vi "Calibration Models Comparison.vi"() -> ()   [LabVIEW 2014]
doc: "This example compares measurement accuracies obtained using different types of calibration models. Several calibration templates have been learned offline using the Calibration Training interface.\n\nFor each of the calibration models, the example locates the part in the image and measures its height along 50 search lines. The process is repeated for 25 different locations in the image using the same part. The example computes the average and standard deviation of the measurement set and plots the measurement distribution in a histogram."
uses:
  <vilib>/Utility/miscctls.llb/LVRowAndColumnUnsignedTypeDef.ctl
  <vilib>/Analysis/NI_AALBase.lvlib
  <vilib>/vision/NI_Vision_Development_Module.lvlib
panel:
  in  "Tab Control":enum32{"Part Image", "Calibration Grid Image"}(tab)
  out "Test Image":T1(plugin-control)
  out "Calibration Grid":T1(plugin-control)
  in  "Stop Button":bool
  out "Measurement Distribution Graph":T2(graph)
  in  "Results":i32(listbox)
  # "Overview: Compares accuracy and speed of the different spatial calibration methods.\nRequirements: NI Vision Development Module\nInstructions: Run the VI."
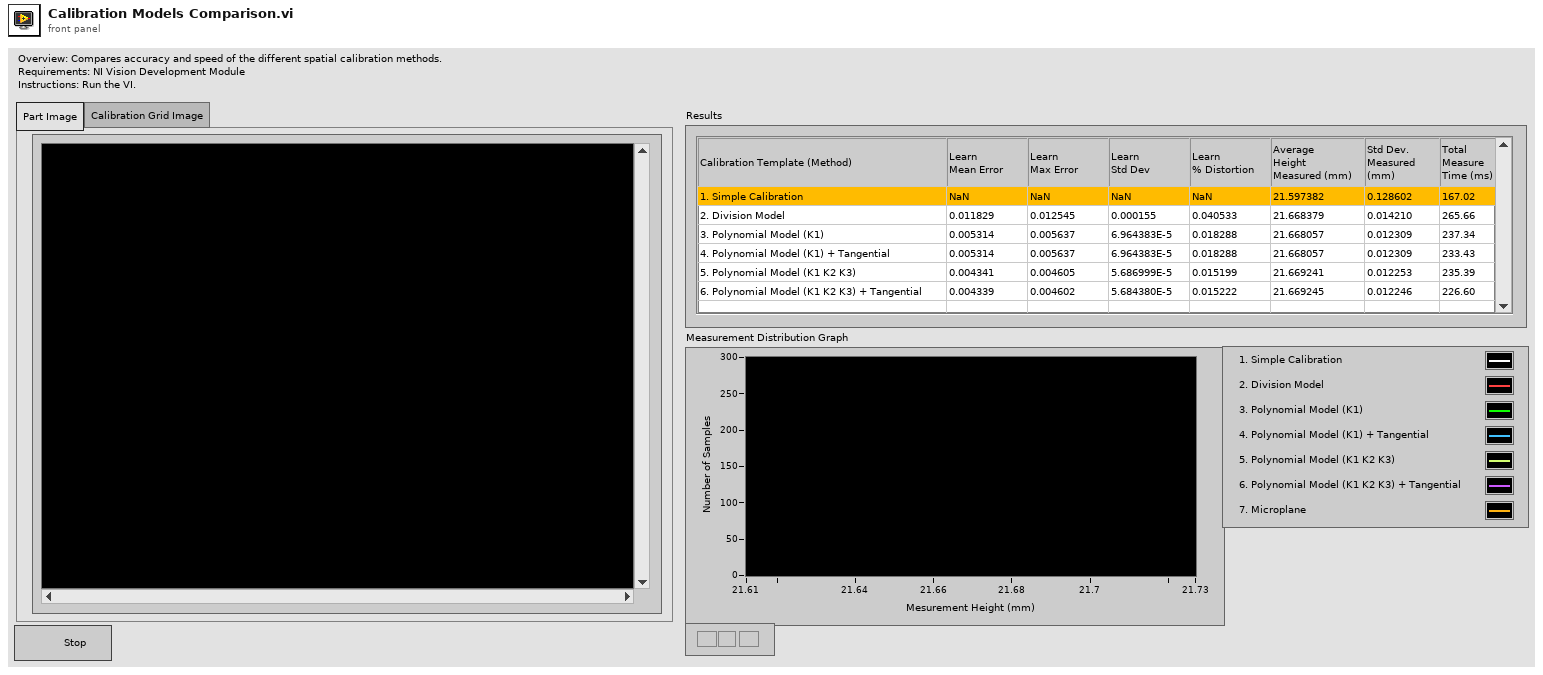
[diagram p1: front panel]
types:
  T1 = typedef "IMAQ Image.ctl" = refnum<image>
  T2 = cluster{"X Values":dbl[], "Histogram: h(x)":i32[]}[]
  T3 = typedef "LVRowAndColumnUnsignedTypeDef.ctl" = cluster{"Row":u32, "Column":u32}
  T4 = typedef "Correction Learn Setup.ctl" = cluster{"Method":u32, "Distortion":T5, "Corrected Image Scaling":u32, "Corrected Image Learn ROI":u32, "Learn Correction Table?":bool}
  T5 = typedef "Distortion Model Types.ctl" = i32
  T6 = typedef "Error Statistics.ctl" = cluster{"Mean Error":dbl, "Maximum Error":dbl, "Standard Deviation":dbl, "% Distortion":dbl}
  T7 = cluster{"X Values":dbl[], "Histogram: h(x)":i32[]}
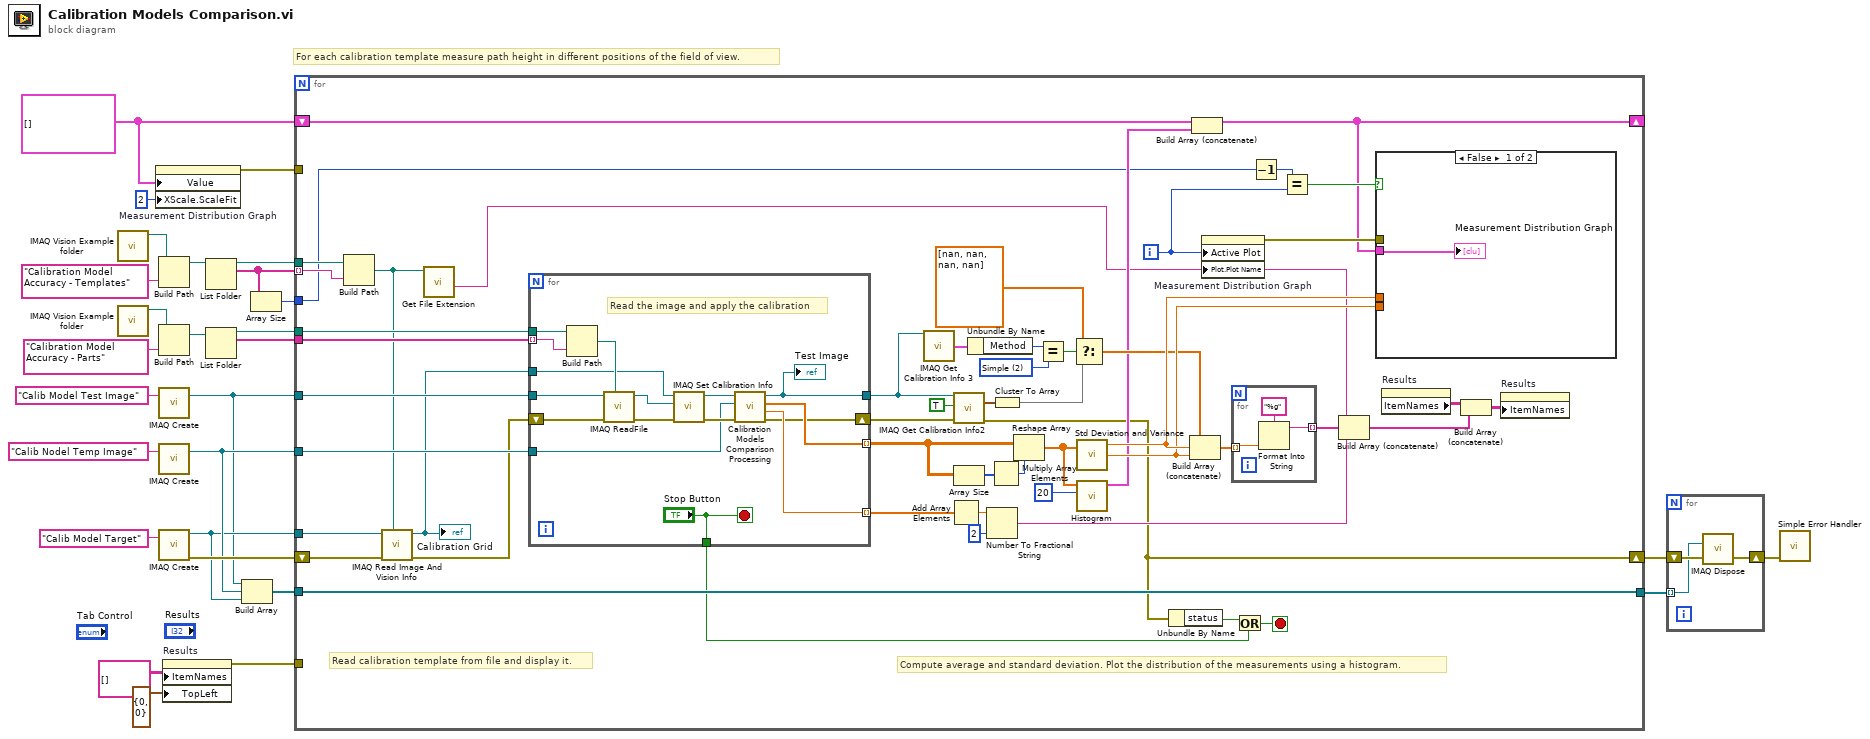
[diagram p0: block diagram]
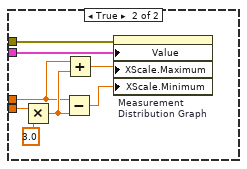
[diagram p2: hidden frame]
diagram:
  w17 = T2 [] ("Measurement Distribution")
  # "For each calibration template measure path height in different positions of the field of view."
  n1 = call "IMAQ Vision Example folder.vi"() -> ("Example Image Path"=w14:path)  [unwired: 11 in]
  n2 = call "IMAQ Vision Example folder.vi"() -> ("Example Image Path"=w12:path)  [unwired: 11 in]
  n3 = property on="Measurement Distribution Graph" class="XYGraph (strict)"("Value"=w17, "XScale.ScaleFit"=u8 2 ("X Scale.Scale Fit")) -> (error out=w16:errorcluster)  [unwired: 2 in, 1 out]
  n4 = Build Path(base path=w14, name or relative path="Calibration Model Accuracy - Templates") -> (appended path=w13:path)
  n5 = Build Path(base path=w12, name or relative path="Calibration Model Accuracy - Parts") -> (appended path=w11:path)
  n6 = call "IMAQ Create"("Image Name"="Calib Model Test Image") -> ("New Image"=w6:T1)  [unwired: 3 in, 2 out]
  n7 = call "IMAQ Create"("Image Name"="Calib Nodel Temp Image") -> ("New Image"=w9:T1)  [unwired: 3 in, 2 out]
  n8 = call "IMAQ Create"("Image Name"="Calib Model Target") -> ("New Image"=w8:T1, "error out"=w23:errorcluster)  [unwired: 3 in, 1 out]
  n9 = property on="Results" class="MCListbox (strict)"("ItemNames"=string[][] [] ("Item Names"), "TopLeft"=T3 {"Row"=0, "Column"=0} ("Top Left Visible Cell")) -> (error out=w20:errorcluster)  [unwired: 2 in, 1 out]
  n10 = List Folder(path=w13) -> (path out=w22:path, filenames=w2:string[])  [unwired: 1 in, 4 out]
  n11 = List Folder(path=w11) -> (path out=w27:path, filenames=w26:string[])  [unwired: 1 in, 4 out]
  n12 = Build Array(w6, w9, w8) -> (w7:T1[])
  n13 = Array Size(array=w2) -> (size(s)=w1:i32)
  n14 = for {
    tunnel: w27 -> [w77]
    tunnel: w26 -> [w76]
    tunnel: w6 -> [w75]
    tunnel: w9 -> [w74]
    tunnel: w8 -> [w80]
    tunnel: w22 -> [w78]
    tunnel: w2 -> [w72] mode=indexing
    tunnel: w20 -> [_]
    shift-right: [w50] -> _
    shift-left: w17 -> [w70]
    tunnel: w16 -> [_]
    shift-right: [w35] -> w5
    shift-left: w23 -> [w79]
    tunnel: w7 -> [w47]
    tunnel: [w47] -> w4
    tunnel: w1 -> [w36]
    i -> [w71]
    stop <- w33 stop-if-true
    w42 = u32 2 items=["Perspective", "Microplane", "Simple", "Corrected", "None"] ("Method")
    # "Compute average and standard deviation. Plot the distribution of the measurements using a histogram."
    # "Read calibration template from file and display it."
    n15 = Build Path(base path=w78, name or relative path=w72) -> (appended path=w31:path)
    n16 = call "IMAQ Read Image And Vision Info"("File Path"=w31, "error in (no error)"=w79, "Image"=w80) -> ("error out"=w73:errorcluster, "Image Out"=w48:T1)  [unwired: 1 in, 6 out]
    "Calibration Grid" <- w48
    n17 = call <vilib>:"Get File Extension.vi"("file"=w31) -> ("filename without extension"=w30:string)  [unwired: 7 in, 3 out]
    n18 = for {
      tunnel: w77 -> [w108]
      tunnel: w76 -> [w107] mode=indexing
      tunnel: w75 -> [w106]
      tunnel: w74 -> [w93]
      tunnel: [w104] -> w46 mode=indexing
      tunnel: w48 -> [w97]
      tunnel: ["Stop Button"] -> w32
      tunnel: [w103] -> w68 mode=indexing
      shift-right: [w94] -> w49
      shift-left: w73 -> [w100]
      tunnel: [w95] -> w45
      stop <- "Stop Button" stop-if-true
      # "Read the image and apply the calibration"
      n19 = Build Path(base path=w108, name or relative path=w107) -> (appended path=w105:path)
      n20 = call "IMAQ ReadFile"("File Path"=w105, "error in (no error)"=w100, "Image"=w106) -> ("error out"=w99:errorcluster, "Image Out"=w101:T1)  [unwired: 2 in, 5 out]
      n21 = call "IMAQ Set Calibration Info"("error in (no error)"=w99, "Image Dst"=w101, "Image Src"=w97) -> ("error out"=w98:errorcluster, "Calibrated Image"=w96:T1)  [unwired: 1 in, 6 out]
      n22 = call "Calibration Models Comparison Processing.vi"("error in (no error)"=w98, "Temp Image"=w93, "Test Image"=w96) -> ("error out"=w94:errorcluster, "Elapsed Time (ms)"=w103:dbl, "Results"=w104:sgl[], "Test Image Out"=w95:T1)  [unwired: 5 in]
      "Test Image" <- w95
    }
    n23 = call "IMAQ Get Calibration Info 3"("Calibration Template Image"=w45) -> ("Calibration Learn Setup"=w44:T4)  [unwired: 6 in, 8 out]
    n24 = Add Array Elements(numeric array=w68) -> (sum=w69:dbl)
    n25 = call "IMAQ Get Calibration Info2"("Calibration Template Image"=w45, "Return Error Information (False)"=TRUE, "error in (no error)"=w49) -> ("Error Statistics"=w65:T6, "error out"=w35:errorcluster)  [unwired: 11 out]
    n26 = Array Size(array=w46) -> (size(s)=w67:i32[])
    n27 = Unbundle By Name(w44) -> ("Method"=w43:u32)
    n28 = Number To Fractional String(number=w69, precision (6)=i16 2) -> (F-format string=w51:string)  [unwired: 2 in]
    n29 = Multiply Array Elements(1:w67) -> (0:w59:i32)
    n30 = Cluster To Array(cluster=w65) -> (array=w40:dbl[])
    n31 = Reshape Array(w46, w59) -> (w57:sgl[])
    n32 = Equal?(x=w43, y=w42) -> (x = y?=w41:bool)
    n33 = Select(t=dbl[] [nan, nan, nan, nan], s=w41, f=w40) -> (s? t:f=w39:dbl[])
    n34 = call <vilib>:"Std Deviation and Variance.vi"("X"=w57) -> ("mean"=w53:dbl, "standard deviation"=w52:dbl)  [unwired: 1 in, 1 out]
    n35 = call <vilib>:"Histogram.vi"("intervals"=20, "X"=w57) -> ("Histogram Graph"=w37:T7)  [unwired: 9 out]
    n36 = Unbundle By Name(w35) -> ("status"=w34:bool)
    n37 = Build Array (concatenate)(w39, w53, w52) -> (w62:dbl[])
    n38 = Build Array (concatenate)(w70, w37) -> (w50:T2)
    n39 = property on="Measurement Distribution Graph" class="XYGraph (strict)"("Active Plot"=w71, "Plot.Plot Name"=w30) -> (error out=w58:errorcluster)  [unwired: 2 in, 1 out]
    n40 = for {
      tunnel: w62 -> [w92] mode=indexing
      tunnel: [w90] -> w54 mode=indexing
      n41 = Format Into String(format string="%g", w92) -> (resulting string=w90:string)  [unwired: 2 in, 1 out]
    }
    n42 = Or(x=w34, y=w32) -> (x .or. y?=w33:bool)
    n43 = Decrement(x=w36) -> (x-1=w55:i32)
    n44 = Equal?(x=w55, y=w71) -> (x = y?=w56:bool)
    n45 = Build Array (concatenate)(w30, w54, w51) -> (w61:string[])
    n46 = case shown="False" w56 {
      tunnel: w58 -> [_ w89]
      tunnel: w53 -> [_ w86]
      tunnel: w52 -> [_ w88]
      tunnel: w50 -> [w81 w82]
      frame False {
        "Measurement Distribution Graph" <- w81
      }
      frame True {
        n47 = Multiply(x=w88, y=3.0) -> (x*y=w87:dbl)
        n48 = Subtract(x=w86, y=w87) -> (x-y=w84:dbl)
        n49 = Add(x=w86, y=w87) -> (x+y=w83:dbl)
        n50 = property on="Measurement Distribution Graph" class="XYGraph (strict)"(error in=w89, "Value"=w82, "XScale.Maximum"=w83, "XScale.Minimum"=w84) -> ()  [unwired: 1 in, 2 out]
      }
    }
    n51 = property on="Results" class="MCListbox (strict)"() -> ("ItemNames"=w64:string[][])  [unwired: 2 in, 2 out]
    n52 = Build Array (concatenate)(w64, w61) -> (w63:string[][])
    n53 = property on="Results" class="MCListbox (strict)"("ItemNames"=w63) -> ()  [unwired: 2 in, 2 out]
  }
  n54 = for {
    tunnel: w4 -> [w110] mode=indexing
    shift-right: [w109] -> w3
    shift-left: w5 -> [w111]
    n55 = call "IMAQ Dispose"("Image"=w110, "error in (no error)"=w111) -> ("error out"=w109:errorcluster)  [unwired: 4 in]
  }
  n56 = call <vilib>:"Simple Error Handler.vi"("error in (no error)"=w3) -> ()  [unwired: 4 in, 5 out]
